vi "configure.vi"(8 "error in (no error)":errorcluster, 11 "GenericPlugin in":refnum<class "FPGAWrapperDL090211Galvo.lvclass">) -> (0 "error out":errorcluster, 3 "GenericPlugin out":refnum<class "FPGAWrapperDL090211Galvo.lvclass">)   [LabVIEW 2010, in "FPGAWrapperDL090211Galvo.lvclass"]
doc: "The dynamic dispatch version of this VI loads and displays the configuration file associated with the plug-in object. The user modify and save the configuration data."
uses:
  FPGAWrapperDL090211Galvo.lvclass
  type definitions/bit_file_enum.ctl
  FPGAWrapperDL090211Galvo.lvclass/FPGAWrapperDL090211Galvo.ctl
  common/classes/GenericComponent/GenericComponent/GenericComponent.lvclass
panel:
  in  "bit file":T1
  in  "ADC clock phase delay":i32=1 min=1 max=2
  out "configuration":string
  in  "cancelButton":bool
  in  "okButton":bool
  in  "HIFO ADC version":i32=1 min=1 max=2
  # "Configure FPGAWrapperDL090211Galvo_grabber"
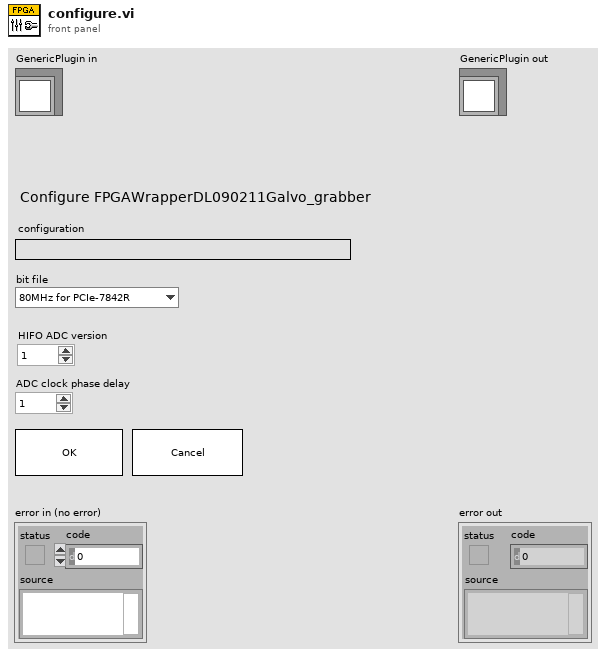
[diagram p1: front panel]
types:
  T1 = typedef "bit_file_enum.ctl" = enum16{"80MHz for PCIe-7842R", "120MHz for PCIe-7842R"}
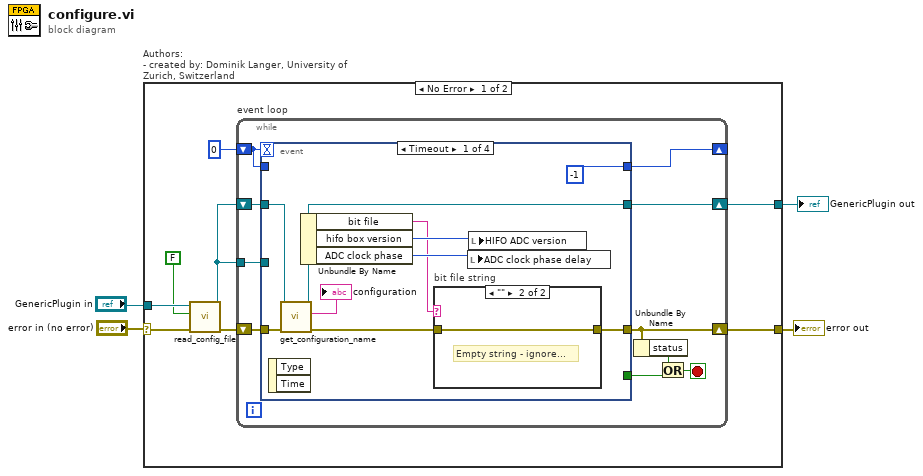
[diagram p0: block diagram]
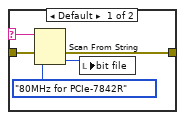
[diagram p2: hidden frame]
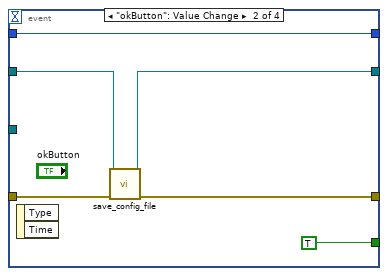
[diagram p3: hidden frame]
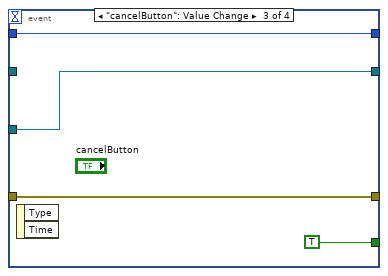
[diagram p4: hidden frame]
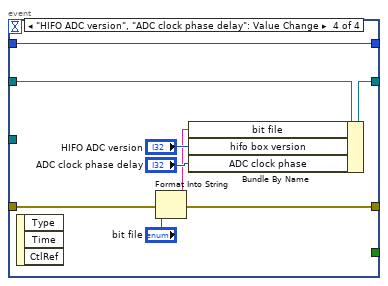
[diagram p5: hidden frame]
diagram:
  n1 = case "Authors: \n- created by: Dominik Langer, University of Zurich, Switzerland" shown="No Error" "error in (no error)" {
    selector: "error in (no error)" -> [w12 w58]
    tunnel: "GenericPlugin in" -> [w10 w59]
    tunnel: [w7 w58] -> w2
    tunnel: [w6 w59] -> w1
    frame No Error {
      n2 = call-dynamic "read_config_file.vi"("error in (no error)"=w12, "force load?"=FALSE, "GenericPlugin in"=w10) -> ("error out"=w11:errorcluster, "GenericPlugin out"=w8:refnum<class "FPGAWrapperDL090211Galvo.lvclass">)  [unwired: 7 in]
      n3 = while "event loop" {
        shift-right: [w18] -> w7
        shift-left: w11 -> [w21]
        shift-right: [w20] -> w6
        shift-left: w8 -> [w22]
        tunnel: w8 -> [w19]
        shift-right: [w13] -> _
        shift-left: 0 -> [w14]
        stop <- w15 stop-if-true
        n4 = event shown="[0] Timeout" {
          selector: _ -> [_ _ _ _]
          dyn-events: _ -> [_ _ _ _]
          timeout: w14 -> [_ _ _ _]
          tunnel: w22 -> [w30 w42 _ w57]
          tunnel: w21 -> [w31 w44 w48 w52]
          tunnel: [w24 w43 w48 w51] -> w18
          tunnel: [w29 w41 w47 w56] -> w20
          tunnel: w19 -> [_ _ w47 _]
          tunnel: [_ TRUE TRUE _] -> w16
          tunnel: w14 -> [_ w39 w45 w53]
          tunnel: [-1 w39 w45 w53] -> w13
          event Timeout {
            n5 = event-data() -> ()  [unwired: 1 in, 2 out]
            n6 = call "get_configuration_name.vi"("error in (no error)"=w31, "GenericPlugin.lvclass in"=w30) -> ("error out"=w25:errorcluster, "configuration name"=→"configuration":string, "GenericPlugin.lvclass out"=w29:refnum<class "FPGAWrapperDL090211Galvo.lvclass">)  [unwired: 7 in]
            n7 = Unbundle By Name(w29) -> ("bit file"=w23:string, "hifo box version"=w32:i32, "ADC clock phase"=w27:i32)
            n8 = case "bit file string" shown="\"\"" w23 {
              selector: w23 -> [w33 _]
              tunnel: w25 -> [w37 w38]
              tunnel: [w36 w38] -> w24
              frame Default {
                n9 = Scan From String(input string=w33, error in=w37, default 1=bit_file_enum."80MHz for PCIe-7842R" ("bit file")) -> (error out=w36:errorcluster, output 1=w34:T1)  [unwired: 2 in, 2 out]
                n10 = local write "bit file"(w34) -> ()
              }
              frame "" {
                # "Empty string - ignore..."
              }
            }
            n11 = local write "ADC clock phase delay"(w27) -> ()
            n12 = local write "HIFO ADC version"(w32) -> ()
          }
          event "okButton": Value Change {
            n13 = event-data() -> ()  [unwired: 1 in, 2 out]
            n14 = call-dynamic "save_config_file.vi"("error in (no error)"=w44, "GenericPlugin in"=w42) -> ("error out"=w43:errorcluster, "GenericPlugin out"=w41:refnum<class "FPGAWrapperDL090211Galvo.lvclass">)  [unwired: 8 in]
          }
          event "cancelButton": Value Change {
            n15 = event-data() -> ()  [unwired: 1 in, 2 out]
          }
          event "HIFO ADC version", "ADC clock phase delay": Value Change {
            n16 = event-data() -> ()  [unwired: 1 in, 3 out]
            n17 = Format Into String(error in=w52, "bit file") -> (resulting string=w49:string, error out=w51:errorcluster)  [unwired: 2 in]
            n18 = Bundle By Name(cluster=w57, "bit file"=w49, "hifo box version"="HIFO ADC version", "ADC clock phase"="ADC clock phase delay") -> (w56:refnum<class "FPGAWrapperDL090211Galvo.lvclass">)
          }
        }
        n19 = Unbundle By Name(w18) -> ("status"=w17:bool)
        n20 = Or(x=w17, y=w16) -> (x .or. y?=w15:bool)
      }
    }
    frame Error {
    }
  }
  "error out" <- w2
  "GenericPlugin out" <- w1
